vi "Voltage (with Events) - Continuous Input.vi"() -> ()   [LabVIEW 2022 SP3]
doc: "This example demonstrates how to continuously acquire buffered voltage measurements using a DAQmx device. It uses software events to ensure that the program does not become unresponsive while waiting for samples to become available.\n\nFor instructions on how to connect your signals to the DAQ device, refer to your device documentation."
uses:
  <vilib>/Utility/error.llb/DialogType.ctl
  <vilib>/DAQmx/read.llb/DAQmx Read (Analog 1D Wfm NChan NSamp).vi
  <vilib>/DAQmx/create/channels.llb/DAQmx Create Channel (AI-Voltage-Basic).vi
  <vilib>/DAQmx/configure/timing.llb/DAQmx Timing (Sample Clock).vi
  <vilib>/DAQmx/configure/task.llb/DAQmx Configure Logging (TDMS).vi
  <vilib>/DAQmx/configure/trigger.llb/DAQmx Start Trigger (Digital Edge).vi
  <vilib>/DAQmx/configure/trigger.llb/DAQmx Start Trigger (Time).vi
  <vilib>/DAQmx/configure/trigger.llb/DAQmx Start Trigger (Analog Edge).vi
  <vilib>/DAQmx/miscellaneous.llb/DAQmx Fill In Error Info.vi
  <resource>/objmgr/daqmx.rc
panel:
  in  "Samples per File":i32=100
  in  "Group Name":string
  in  "Trigger Type":T1(tab)
  in  "Digital Start Trigger Edge":i32(ring)=10280 caption="Edge" items=["Rising"=10280, "Falling"=10171]
  in  "Digital Start Trigger Source":tag="/Dev1/PFI0" caption="Source"
  in  "Digital Pause Trigger Pause When":i32(ring)=10192 caption="Pause When" items=["High"=10192, "Low"=10214]
  in  "Digital Pause Trigger Source":tag="/Dev1/PFI0" caption="Source"
  in  "Analog Start Trigger Level":dbl caption="Level" format="%0.2f"
  in  "Analog Start Trigger Hysteresis":dbl caption="Hysteresis" format="%.2f"
  in  "Analog Start Trigger Slope":i32(ring)=10280 caption="Slope" items=["Rising"=10280, "Falling"=10171]
  in  "Analog Start Trigger Source":string="APFI0" caption="Source"
  in  "Analog Pause Trigger Source":string="APFI0" caption="Source"
  in  "Analog Pause Trigger Pause When":i32(ring)=10093 caption="Pause When" items=["Above Level"=10093, "Below Level"=10107]
  in  "Analog Pause Trigger Level":dbl caption="Level" format="%.2f"
  in  "When":timestamp
  in  "Select Time\nManually":bool
  in  "Stop":bool
  out "Waveform Graph":waveform(dbl)[](graph)
  in  "TDMS File Path":path
  in  "Samples per Loop":i32=100
  in  "Sample Rate":dbl=1000.0
  in  "Sample Clock Source":tag="OnboardClock"
  in  "Terminal Configuration":i32(ring)=-1 items=["default"=-1, "RSE"=10083, "NRSE"=10078, "Differential"=10106, "Pseudodifferential"=12529]
  in  "Max Voltage":dbl=5.0
  in  "Min Voltage":dbl=-5.0
  in  "Physical Channel":tag="Dev1/ai0"
  out "Actual Sample Rate":dbl format="%0.2f"
  in  "Logging Mode":i32(ring)=10231 items=["Off"=10231, "Log and Read"=15842]
  # "Channel Settings"
  # "Acquired Data"
  # "Timing Settings"
  # "Trigger Settings"
  # "Logging Settings"
  # "To enable triggers, select a tab above, and configure the settings.\n\nNot all hardware supports all trigger types. Refer to your device documentation for more information."
  # "This trigger type is not supported in continuous sample timing. \n\nRefer to your device documentation for more information on which triggers are supported."
  # "This trigger type is not supported in continuous sample timing. \n\nRefer to your device documentation for more information on which triggers are supported."
  # "If time is not manually set, task will begin after 10 seconds"
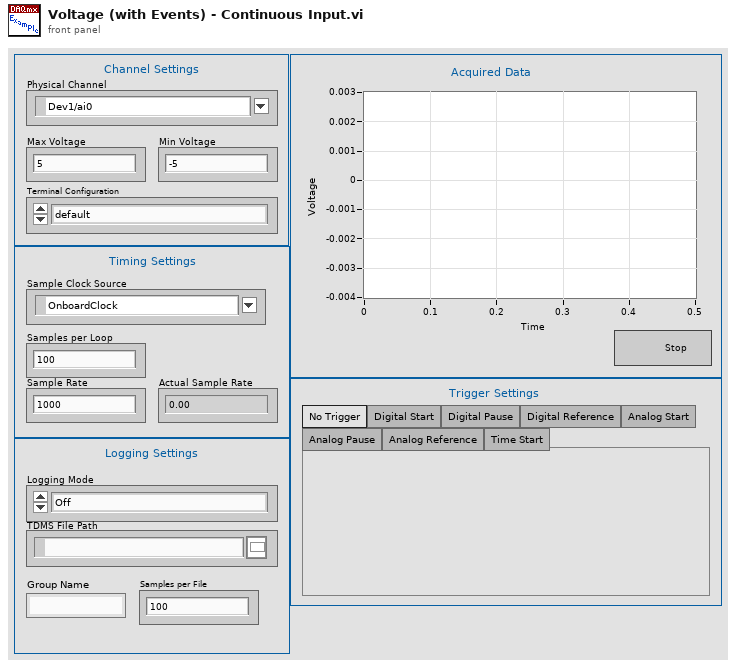
[diagram p1: front panel]
types:
  T1 = enum32{"No Trigger", "Digital Start", "Digital Pause", "Digital Reference", "Analog Start", "Analog Pause", "Analog Reference", "Time Start"}
  T2 = typedef "DialogType.ctl" = u16
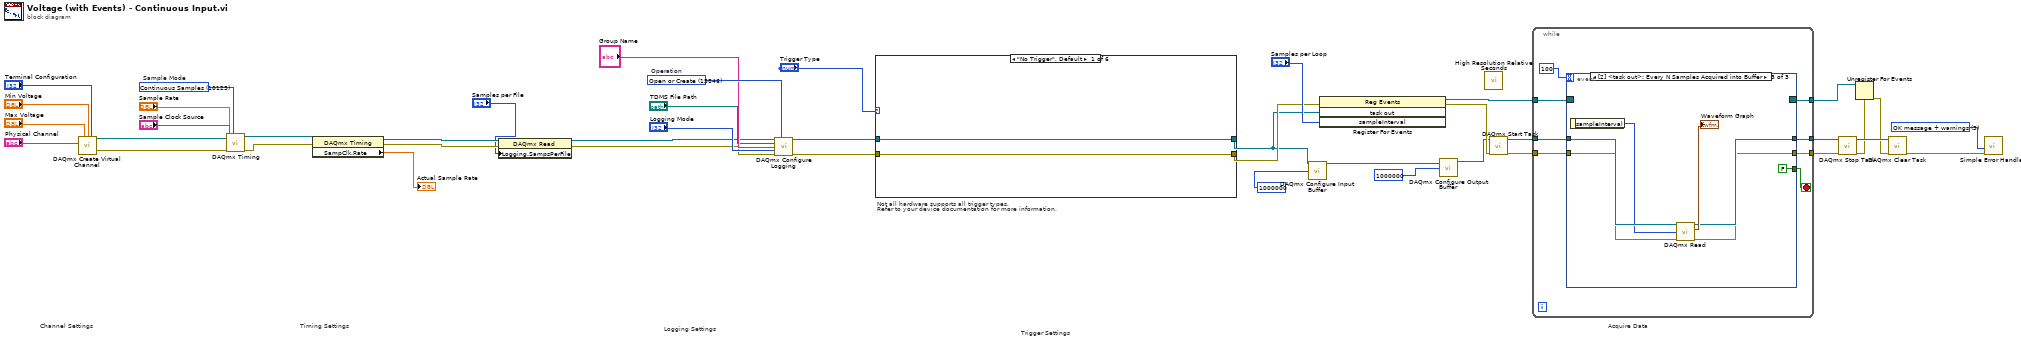
[diagram p0: block diagram]
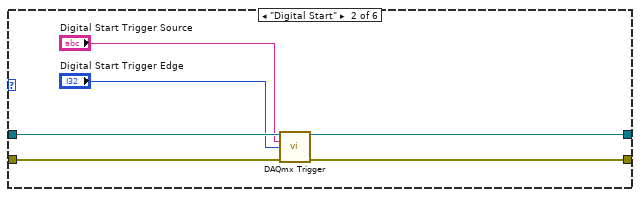
[diagram p2: hidden frame]
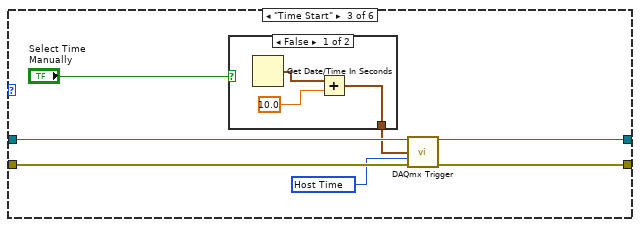
[diagram p3: hidden frame]
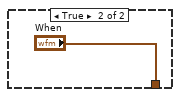
[diagram p4: hidden frame]
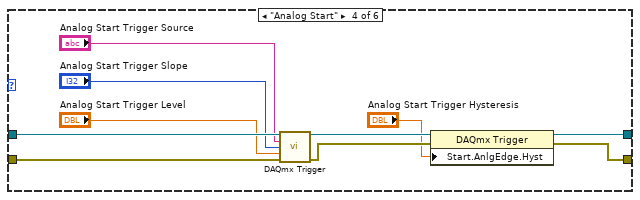
[diagram p5: hidden frame]
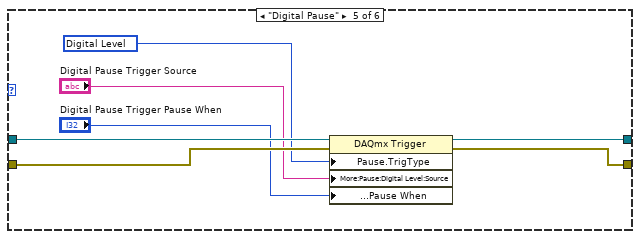
[diagram p6: hidden frame]
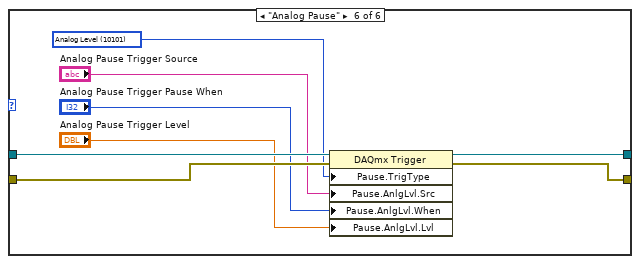
[diagram p7: hidden frame]
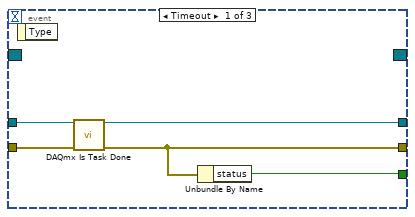
[diagram p8: hidden frame]
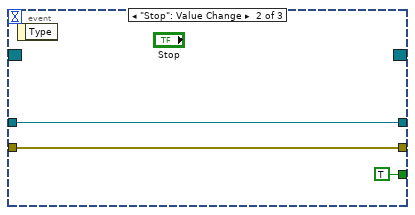
[diagram p9: hidden frame]
diagram:
  w23 = T2 3 items=["no dialog", "OK message", "continue or stop message", "OK message + warnings", "continue/stop + warnings"] ("type of dialog (OK msg:1)")
  w38 = 15846 items=["Open"=10437, "Open or Create"=15846, "Create or Replace"=15847, "Create"=15848]  # Operation
  w41 = 10123 items=["Finite Samples"=10178, "Continuous Samples"=10123, "Hardware Timed Single Point"=12522]  # Sample Mode
  # "Trigger Settings"
  # "Not all hardware supports all trigger types.\nRefer to your device documentation for more information."
  # "Acquire Data"
  # "Logging Settings"
  # "Timing Settings"
  # "Channel Settings"
  n1 = call-poly <vilib>:"DAQmx Create Virtual Channel.vi"("maximum value"="Max Voltage", "minimum value"="Min Voltage", "input terminal configuration"="Terminal Configuration", "physical channels"="Physical Channel") -> ("task out"=w39:refnum<k21>, "error out"=w40:errorcluster)  [unwired: 10 in]
  n2 = call-poly <vilib>:"DAQmx Timing.vi"("task/channels in"=w39, "sample mode"=w41, "rate"="Sample Rate", "source"="Sample Clock Source", "error in"=w40) -> ("task out"=w43:refnum<k21>, "error out"=w42:errorcluster)  [unwired: 9 in]
  n3 = property class="DAQmx Timing"(reference=w43, error in=w42) -> (reference out=w13:refnum<k21>, error out=w11:errorcluster, "SampClk.Rate"=→"Actual Sample Rate":dbl)
  n4 = property class="DAQmx Read"(reference=w13, error in=w11, "Logging.SampsPerFile"="Samples per File") -> (reference out=w12:refnum<k21>, error out=w10:errorcluster)
  n5 = call-poly <vilib>:"DAQmx Configure Logging.vi"("task/channels in"=w12, "operation"=w38, "file path"="TDMS File Path", "group name"="Group Name", "logging mode"="Logging Mode", "error in"=w10) -> ("task out"=w17:refnum<k21>, "error out"=w16:errorcluster)  [unwired: 8 in]
  n6 = case shown="\"No Trigger\", Default" "Trigger Type" {
    tunnel: w17 -> [w45 w51 w58 w72 w79 w87]
    tunnel: w16 -> [w44 w50 w57 w71 w76 w84]
    tunnel: [w45 w49 w56 w69 w78 w86] -> w5
    tunnel: [w44 w48 w55 w68 w77 w85] -> w18
    frame "No Trigger", Default {
    }
    frame "Digital Start" {
      n7 = call-poly <vilib>:"DAQmx Trigger.vi"("task/channels in"=w51, "source"="Digital Start Trigger Source", "edge"="Digital Start Trigger Edge", "error in"=w50) -> ("task out"=w49:refnum<k21>, "error out"=w48:errorcluster)  [unwired: 10 in]
    }
    frame "Time Start" {
      w54 = 16126 items=["Host Time"=16126, "I/O Device Time"=16127] ("timescale")
      n8 = case shown="False" "Select Time\nManually" {
        tunnel: [w60 "When"] -> w52
        frame False {
          n9 = Get Date/Time In Seconds() -> (seconds since 1Jan1904=w61:timestamp)
          n10 = Add(x=w61, y=10.0) -> (x+y=w60:timestamp)
        }
        frame True {
        }
      }
      n11 = call-poly <vilib>:"DAQmx Trigger.vi"("task/channels in"=w58, "when"=w52, "timescale"=w54, "error in"=w57) -> ("task out"=w56:refnum<k21>, "error out"=w55:errorcluster)  [unwired: 10 in]
    }
    frame "Analog Start" {
      n12 = call-poly <vilib>:"DAQmx Trigger.vi"("task/channels in"=w72, "source"="Analog Start Trigger Source", "slope"="Analog Start Trigger Slope", "level"="Analog Start Trigger Level", "error in"=w71) -> ("task out"=w67:refnum<k21>, "error out"=w66:errorcluster)  [unwired: 9 in]
      n13 = property class="DAQmx Trigger"(reference=w67, error in=w66, "Start.AnlgEdge.Hyst"="Analog Start Trigger Hysteresis") -> (reference out=w69:refnum<k21>, error out=w68:errorcluster)
    }
    frame "Digital Pause" {
      w75 = 10152 items=["Analog Level"=10101, "Analog Window"=10103, "Digital Level"=10152, "Digital Pattern"=10398, "None"=10230] ("Pause.TrigType")
      n14 = property class="DAQmx Trigger"(reference=w79, error in=w76, "Pause.TrigType"=w75, "More:Pause:Digital Level:Source"="Digital Pause Trigger Source", "More:Pause:Digital Level:Pause When"="Digital Pause Trigger Pause When") -> (reference out=w78:refnum<k21>, error out=w77:errorcluster)
    }
    frame "Analog Pause" {
      w83 = 10101 items=["Analog Level"=10101, "Analog Window"=10103, "Digital Level"=10152, "Digital Pattern"=10398, "None"=10230] ("Pause.TrigType")
      n15 = property class="DAQmx Trigger"(reference=w87, error in=w84, "Pause.TrigType"=w83, "Pause.AnlgLvl.Src"="Analog Pause Trigger Source", "Pause.AnlgLvl.When"="Analog Pause Trigger Pause When", "Pause.AnlgLvl.Lvl"="Analog Pause Trigger Level") -> (reference out=w86:refnum<k21>, error out=w85:errorcluster)
    }
  }
  n16 = call <vilib>:"DAQmx Configure Input Buffer.vi"("task/channels in"=w5, "buffer size (in samples per channel)"=u32 1000000) -> ("task out"=w4:refnum<k21>)  [unwired: 12 in, 1 out]
  n17 = register-events(error in=w18, w5, "Samples per Loop") -> (reference out=w29:refnum<event-registration>, error out=w27:errorcluster)  [unwired: 1 in]
  n18 = call <vilib>:"DAQmx Configure Output Buffer.vi"("task/channels in"=w4, "buffer size (in samples per channel)"=u32 1000000) -> ("task out"=w3:refnum<k21>)  [unwired: 12 in, 1 out]
  n19 = call <vilib>:"High Resolution Relative Seconds.vi"() -> ()  [unwired: 1 out]
  n20 = call <vilib>:"DAQmx Start Task.vi"("task/channels in"=w3, "error in"=w27) -> ("task out"=w7:refnum<k21>, "error out"=w8:errorcluster)  [unwired: 12 in]
  n21 = while {
    tunnel: w29 -> [w95]
    tunnel: w8 -> [w94]
    tunnel: w7 -> [w93]
    tunnel: [w92] -> w24
    tunnel: [w91] -> w26
    tunnel: [w90] -> w22
    stop <- w89 stop-if-true
    n22 = event shown="[2] <task out>: Every N Samples Acquired into Buffer" {
      selector: w95 -> [_ _ _]
      dyn-events: [_ _ _] -> w91
      timeout: 100 ("Event Timeout") -> [_ _ _]
      tunnel: w94 -> [w100 w102 w108]
      tunnel: w93 -> [w96 w103 w109]
      tunnel: [w99 w103 w106] -> w92
      tunnel: [w98 w102 w105] -> w90
      tunnel: [w97 TRUE FALSE] -> w89
      event Timeout {
        n23 = event-data() -> ()  [unwired: 1 in, 1 out]
        n24 = call <vilib>:"DAQmx Is Task Done.vi"("task/channels in"=w96, "error in"=w100) -> ("task out"=w99:refnum<k21>, "error out"=w98:errorcluster)  [unwired: 11 in, 1 out]
        n25 = Unbundle By Name(w98) -> ("status"=w97:bool)
      }
      event "Stop": Value Change {
        n26 = event-data() -> ()  [unwired: 1 in, 1 out]
      }
      event Every N Samples Acquired into Buffer {
        n27 = event-data() -> ("sampleInterval"=w107:u32)  [unwired: 1 in]
        n28 = call-poly <vilib>:"DAQmx Read.vi"("task/channels in"=w109, "number of samples per channel"=w107, "error in"=w108) -> ("task out"=w106:refnum<k21>, "data"=→"Waveform Graph":waveform(dbl)[], "error out"=w105:errorcluster)  [unwired: 10 in]
      }
    }
  }
  n29 = call <vilib>:"DAQmx Stop Task.vi"("task/channels in"=w24, "error in"=w22) -> ("task out"=w25:refnum<k21>, "error out"=w21:errorcluster)  [unwired: 12 in]
  n30 = Unregister For Events(event registration refnum=w26, error in=w21) -> (error out=w20:errorcluster)
  n31 = call <vilib>:"DAQmx Clear Task.vi"("task in"=w25, "error in"=w20) -> ("error out"=w37:errorcluster)  [unwired: 13 in]
  n32 = call <vilib>:"Simple Error Handler.vi"("type of dialog (OK msg:1)"=w23, "error in (no error)"=w37) -> ()  [unwired: 3 in, 5 out]
